vi "Newport ITX-D3N Read Write.vi"(8 "error in (no error)":errorcluster, 10 "iTHX Commands":T1="*SRTF", 11 "TCP Network Connection in":refnum<k5>) -> (0 "error out":errorcluster, 1 "In Range?":bool, 2 "Output Data":dbl, 3 "TCP Network Connection out":refnum<k5>)   [LabVIEW 2023]
uses:
  Type Definitions/iTHX.ctl
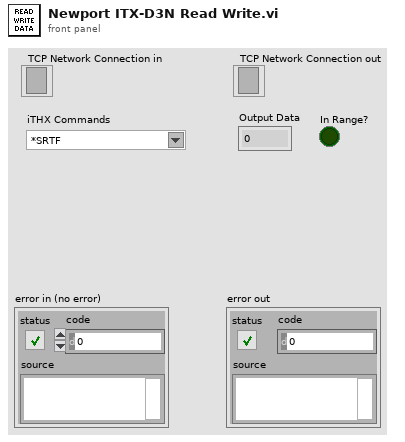
[diagram p1: front panel]
types:
  T1 = typedef "iTHX.ctl" = string
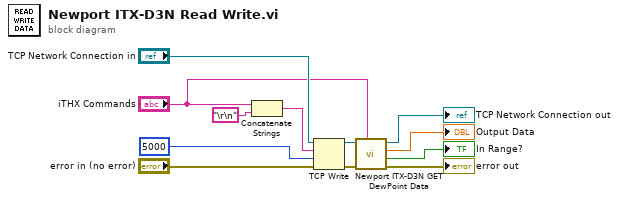
[diagram p0: block diagram]
diagram:
  n1 = Concatenate Strings("iTHX Commands", "\r\n") -> (w10:string)
  n2 = TCP Write(connection ID="TCP Network Connection in", data in=w10, error in (no error)="error in (no error)", 9:5000 ("timeout ms (25000)")) -> (connection ID out=w11:refnum<k5>, error out=w7:errorcluster)  [unwired: 1 out]
  n3 = call "Newport ITX-D3N GET DewPoint Data.vi"("iTHX Commands"="iTHX Commands", "Error In"=w7, "TCP Network Connection In"=w11) -> ("Error Out"=→"error out":errorcluster, "In Range?"=→"In Range?":bool, "Output Data"=→"Output Data":dbl, "TCP Network Connection Out"=→"TCP Network Connection out":refnum<k5>)  [unwired: 5 in]
